vi "ASCIIstringToUnicode.vi"(8 "error in (no error)":errorcluster, 10 "ASCII string":string) -> (0 "error out":errorcluster, 2 "Unicode String":string)   [LabVIEW 2017, in "JKI Simple Localization.lvlib"]
uses:
  API/JKI Simple Localization.lvlib
  kernel32.dll
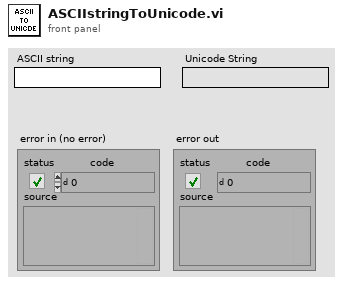
[diagram p1: front panel]
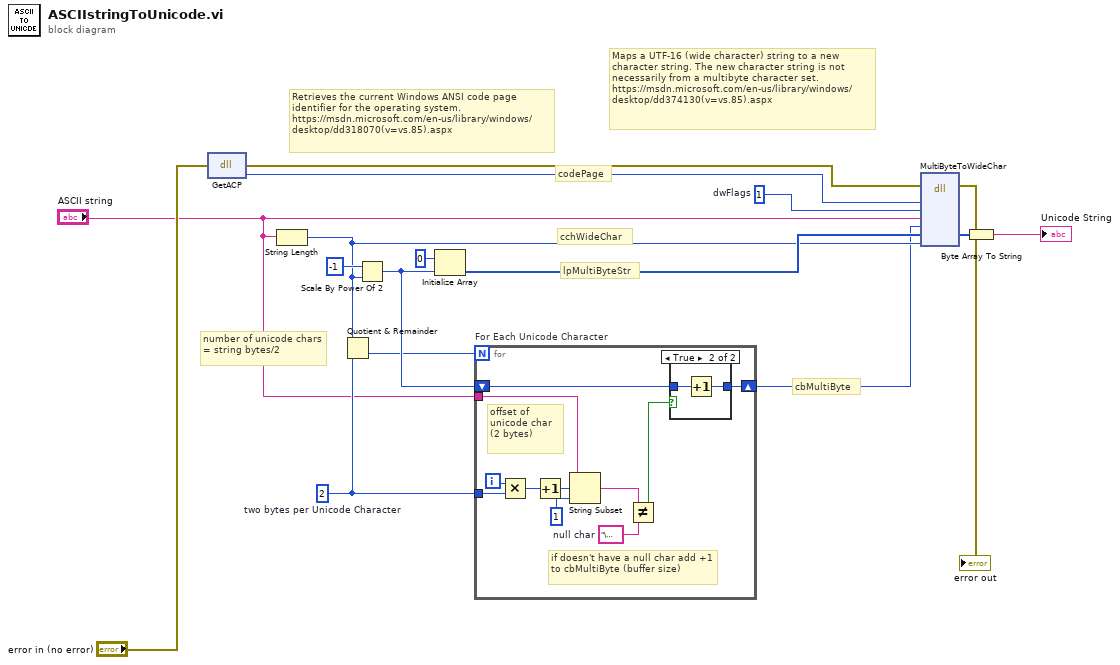
[diagram p0: block diagram]
diagram:
  w11 = 2  # two bytes per Unicode Character
  w8 = u32 1  # dwFlags
  # "Retrieves the current Windows ANSI code page identifier for the operating system.\nhttps://msdn.microsoft.com/en-us/library/windows/desktop/dd318070(v=vs.85).aspx"
  # "codePage"
  # "Maps a UTF-16 (wide character) string to a new character string. The new character string is not necessarily from a multibyte character set.\nhttps://msdn.microsoft.com/en-us/library/windows/desktop/dd374130(v=vs.85).aspx"
  # "cchWideChar"
  # "lpMultiByteStr"
  # "cbMultiByte"
  # "number of unicode chars = string bytes/2"
  n1 = dll-call lib="kernel32.dll" fn="GetACP" label="kernel32.dll\nGetACP"(error in="error in (no error)") -> (error out=w10:errorcluster, w9:u32)  [unwired: 2 in, 1 out]
  n2 = String Length(string="ASCII string") -> (length=w6:i32)
  n3 = Quotient & Remainder(x=w6, y=w11) -> (floor(x/y)=w12:i32)  [unwired: 1 out]
  n4 = Scale By Power Of 2(n=-1, x=w6) -> (x*2^n=w13:i32)
  n5 = Initialize Array(u8 0, w13) -> (w7:u8[])
  n6 = for "For Each Unicode Character" {
    N: w12 -> [_]
    tunnel: w11 -> [w26]
    tunnel: "ASCII string" -> [w24]
    shift-right: [w17] -> w5
    shift-left: w13 -> [w18]
    i -> [w27]
    w20 = "\u0000"  # null char
    # "if doesn't have a null char add +1 to cbMultiByte (buffer size)"
    # "offset of unicode char (2 bytes)"
    n7 = Multiply(x=w27, y=w26) -> (x*y=w25:i32)
    n8 = Increment(x=w25) -> (x+1=w22:i32)
    n9 = String Subset(string=w24, offset (0)=w22, length (rest)=1 ("length (rest)")) -> (substring=w21:string)
    n10 = Not Equal?(x=w21, y=w20) -> (x != y?=w19:bool)
    n11 = case shown="True" w19 {
      tunnel: w18 -> [w28 w30]
      tunnel: [w28 w29] -> w17
      frame False {
      }
      frame True {
        n12 = Increment(x=w30) -> (x+1=w29:i32)
      }
    }
  }
  n13 = dll-call lib="kernel32.dll" fn="MultiByteToWideChar"(error in=w10, "codePage"=w9, "dwFlags"=w8, "pMultiByteStr"="ASCII string", "cbMultiByte"=w5, "lpWideCharStr"=w7, "cchWideChar"=w6) -> (error out=→"error out":errorcluster, "lpWideCharStr"=w4:u8[])  [unwired: 7 in, 2 out]
  n14 = Byte Array To String(unsigned byte array=w4) -> (string=→"Unicode String":string)
